vi "Executable Version.vi"() -> (2 "Version":string)   [LabVIEW 2015, in "Endigit.lvlib"]
doc: "Returns the executable version. If run in the development environment, returns \"Development\".\n\nAuthored by Robert C. Mortensen\nrobert@endigit.com\n\nCopyright (c) 2015, Endigit, Inc."
uses:
  Endigit.lvlib
  version.dll
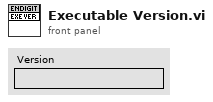
[diagram p1: front panel]
types:
  T1 = enum32{"invalid app kind", "Development System", "Run Time System", "Student Edition", "Embedded LabVIEW", "Evaluation", "Custom"}
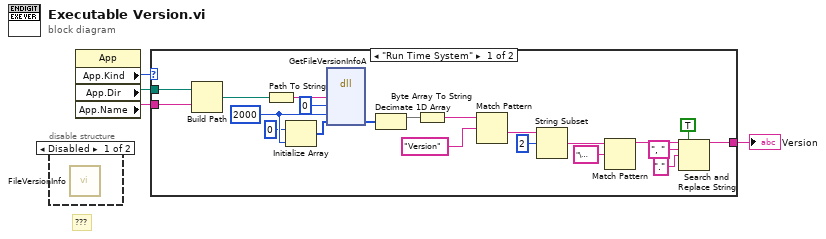
[diagram p0: block diagram]
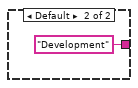
[diagram p3: hidden frame]
diagram:
  # "???"
  n1 = disable-structure shown="Disabled" {
    frame Disabled {
      n2 = call <vilib>:"FileVersionInfo.vi"() -> ()  [unwired: 8 in, 4 out]
    }
    frame Enabled {
    }
  }
  n3 = property class="App"() -> ("App.Kind"=w2:T1, "App.Dir"=w3:path, "App.Name"=w4:string)  [unwired: 2 in, 2 out]
  n4 = case shown="\"Run Time System\"" w2 {
    tunnel: w4 -> [w25 _]
    tunnel: w3 -> [w24 _]
    tunnel: [w5 "Development" ("pattern label")] -> w1
    frame "Run Time System" {
      w13 = u32 2000 ("dwLen")
      n5 = Build Path(base path=w24, name or relative path=w25) -> (appended path=w6:path)
      n6 = Path To String(path=w6) -> (string=w8:string)
      n7 = Initialize Array(u8 0 ("element"), w13) -> (w10:u8[])
      n8 = dll-call lib="version.dll" fn="GetFileVersionInfoA"("lptstrFilename"=w8, "dwHandle"=0, "dwLen"=w13, "lpData"=w10) -> ("lpData"=w11:u8[])  [unwired: 7 in, 2 out]
      n9 = Decimate 1D Array(w11) -> (w12:u8[])  [unwired: 1 out]
      n10 = Byte Array To String(unsigned byte array=w12) -> (string=w14:string)
      n11 = Match Pattern(string=w14, regular expression="Version") -> (after substring=w16:string)  [unwired: 1 in, 3 out]
      n12 = String Subset(string=w16, offset (0)=2) -> (substring=w18:string)  [unwired: 1 in]
      n13 = Match Pattern(string=w18, regular expression="\u0000") -> (before substring=w20:string)  [unwired: 1 in, 3 out]
      n14 = Search and Replace String(replace all?=TRUE ("replace all? (F)"), input string=w20, search string=", ", replace string="." ("replace string (\"\")")) -> (result string=w5:string)  [unwired: 4 in, 3 out]
    }
    frame Default {
    }
  }
  "Version" <- w1
